vi "Pattern Generator.vi"() -> ()   [LabVIEW 2018]
uses:
  Ctls/Protocol Type.ctl
  Interfaces/File Parser Interface.lvlibp/Interfaces/File Parser Interface/File Parser Interface.lvclass
  Interfaces/Protocol Interface.lvlibp/Interfaces/Protocol Interface/Protocol Interface.lvclass
panel:
  out "error out":errorcluster
  in  "stop":bool
  in  "OK Button":bool
  in  "error in":errorcluster
  in  "PinMap":path
  in  "Frequency(Hz)":dbl=0.1 format="%#_13g"
  in  "Wait between Frames(ms)":dbl=1.0 format="%#_13g"
  in  "NumofCycleRd":u32=1
  in  "Protocol Type":T1
  in  "Config File":path
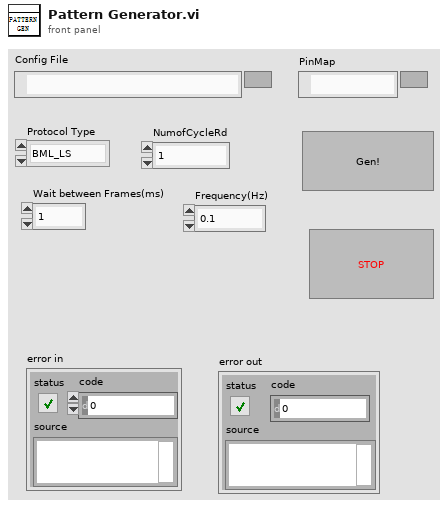
[diagram p1: front panel]
types:
  T1 = typedef "Protocol Type.ctl" = enum16{"BML_LS", "BML_HS", "SPI_3W", "SPI_4W"}
  T2 = cluster{"File Parser Interface.lvclass":refnum<class "File Parser Interface.lvclass">, "Protocol Interface in":refnum<class "Protocol Interface.lvclass">, "Protocol Type":T1, "Config File":path, "Wait between Frames(ms)":dbl, "NumofCycleRd":u32, "PinMap":path, "Frequency(Hz)":dbl}
  T3 = enum16{"init", "wait for input", "Pattern Gen", "error", "end"}
  T4 = typedef "File Parser Interface.lvlibp/Protocol Type.ctl" = enum16{"BML_LS", "BML_HS", "SPI_3W", "SPI_4W"}
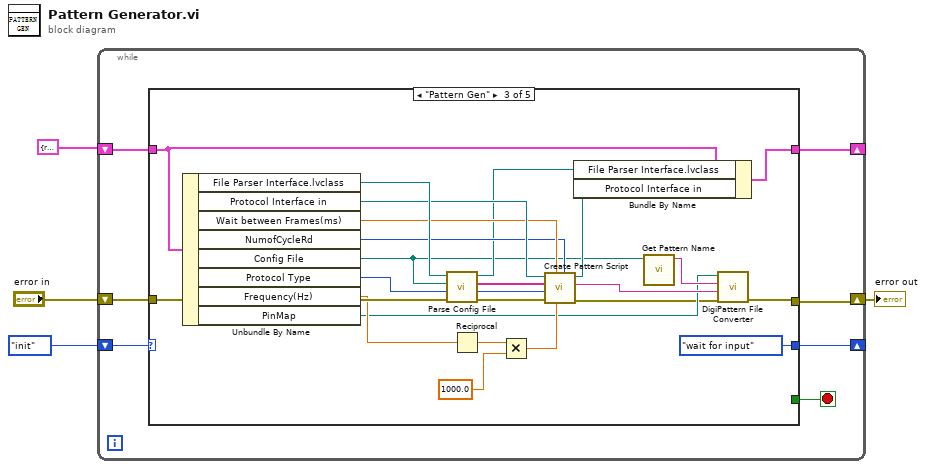
[diagram p0: block diagram]
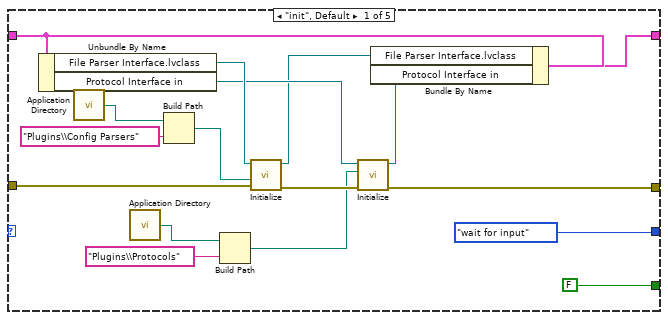
[diagram p2: hidden frame]
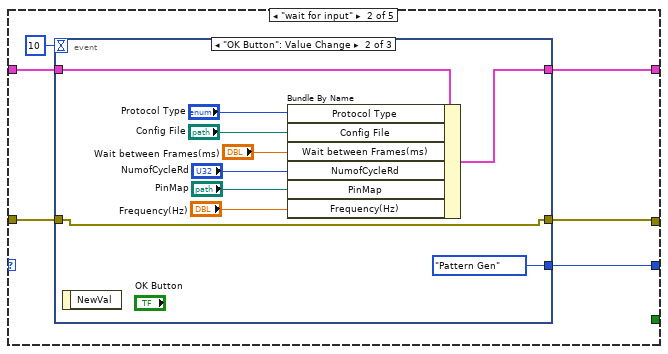
[diagram p3: hidden frame]
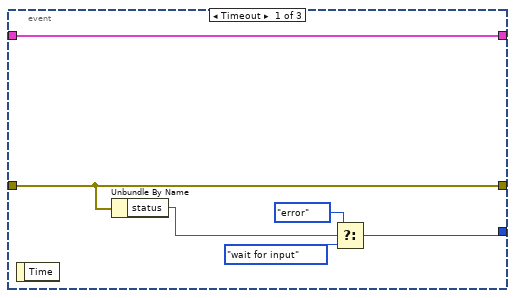
[diagram p4: hidden frame]
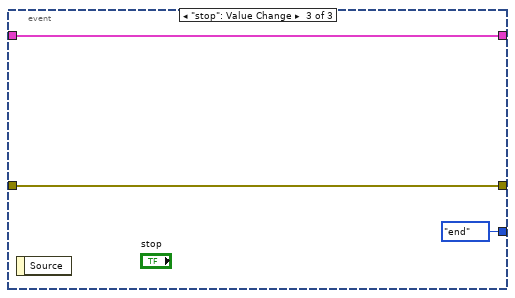
[diagram p5: hidden frame]
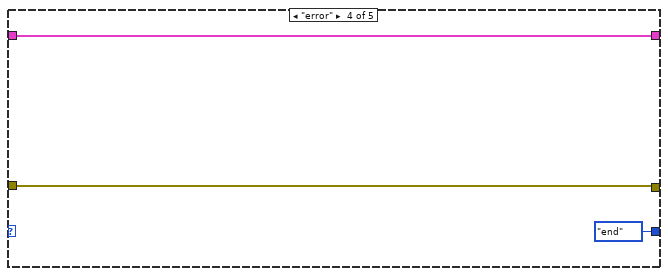
[diagram p6: hidden frame]
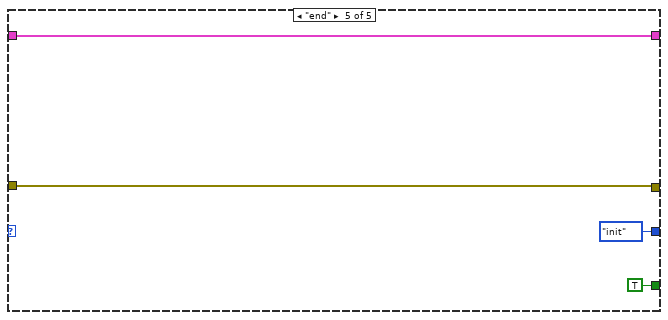
[diagram p7: hidden frame]
diagram:
  n1 = while {
    shift-right: [w10] -> _
    shift-left: T2 {"File Parser Interface.lvclass"=refnum, "Protocol Interface in"=refnum, "Protocol Type"=enum."BML_LS", "Config File"=path "", "Wait between Frames(ms)"=1.0, "NumofCycleRd"=0, "PinMap"=path "", "Frequency(Hz)"=0.0} -> [w11]
    shift-right: [w8] -> w1
    shift-left: "error in" -> [w7]
    shift-right: [w5] -> _
    shift-left: T3."init" -> [w6]
    stop <- w9 stop-if-true
    n2 = case shown="\"Pattern Gen\"" w6 {
      tunnel: w11 -> [w19 w34 w64 w80 w84]
      tunnel: [w16 w33 w61 w80 w84] -> w10
      tunnel: [T3."wait for input" ("f") w29 T3."wait for input" ("f") T3."end" ("f") T3."init" ("f")] -> w5
      tunnel: [FALSE _ _ _ TRUE] -> w9
      tunnel: [w14 w31 w54 w79 w83] -> w8
      tunnel: w7 -> [w13 w32 w77 w79 w83]
      frame "init", Default {
        n3 = Unbundle By Name(w19) -> ("File Parser Interface.lvclass"=w21:refnum<class "File Parser Interface.lvclass">, "Protocol Interface in"=w20:refnum<class "Protocol Interface.lvclass">)
        n4 = call <vilib>:"Application Directory.vi"() -> ("Application Directory"=w27:path)
        n5 = call <vilib>:"Application Directory.vi"() -> ("Application Directory"=w24:path)
        n6 = Build Path(base path=w27, name or relative path="Plugins\\Config Parsers") -> (appended path=w26:path)
        n7 = Build Path(base path=w24, name or relative path="Plugins\\Protocols") -> (appended path=w22:path)
        n8 = call-dynamic "Initialize.vi"("error in (no error)"=w13, "Plugin Folder"=w26, "File Parser Interface in"=w21) -> ("error out"=w25:errorcluster, "File Parser Interface out"=w18:refnum<class "File Parser Interface.lvclass">)  [unwired: 7 in]
        n9 = call "Initialize.vi"("error in (no error)"=w25, "Folder Path"=w22, "Protocol Interface in"=w20) -> ("error out"=w14:errorcluster, "Protocol Interface out"=w17:refnum<class "Protocol Interface.lvclass">)  [unwired: 7 in]
        n10 = Bundle By Name(cluster=w19, "File Parser Interface.lvclass"=w18, "Protocol Interface in"=w17) -> (w16:T2)
      }
      frame "wait for input" {
        n11 = event shown="[1] \"OK Button\": Value Change" {
          selector: _ -> [_ _ _]
          dyn-events: _ -> [_ _ _]
          timeout: 10 -> [_ _ _]
          tunnel: w34 -> [w40 w50 w51]
          tunnel: [w40 w43 w51] -> w33
          tunnel: w32 -> [w39 w42 w53]
          tunnel: [w39 w42 w53] -> w31
          tunnel: [w37 T3."Pattern Gen" T3."end"] -> w29
          event Timeout {
            n12 = event-data() -> ()  [unwired: 1 in, 1 out]
            n13 = Unbundle By Name(w39) -> ("status"=w38:bool)
            n14 = Select(t=T3."error", s=w38, f=T3."wait for input") -> (s? t:f=w37:T3)
          }
          event "OK Button": Value Change {
            n15 = event-data() -> ()  [unwired: 1 in, 1 out]
            n16 = Bundle By Name(cluster=w50, "Protocol Type"="Protocol Type", "Config File"="Config File", "Wait between Frames(ms)"="Wait between Frames(ms)", "NumofCycleRd"="NumofCycleRd", "PinMap"="PinMap", "Frequency(Hz)"="Frequency(Hz)") -> (w43:T2)
          }
          event "stop": Value Change {
            n17 = event-data() -> ()  [unwired: 1 in, 1 out]
          }
        }
      }
      frame "Pattern Gen" {
        n18 = Unbundle By Name(w64) -> ("File Parser Interface.lvclass"=w76:refnum<class "File Parser Interface.lvclass">, "Protocol Interface in"=w74:refnum<class "Protocol Interface.lvclass">, "Wait between Frames(ms)"=w72:dbl, "NumofCycleRd"=w71:u32, "Config File"=w59:path, "Protocol Type"=w69:T1, "Frequency(Hz)"=w68:dbl, "PinMap"=w56:path)
        n19 = call "Parse Config File.vi"("error in (no error)"=w77, "Protocol Type in"=w69, "Config File"=w59, "File Parser Interface in"=w76) -> ("error out"=w75:errorcluster, "Protocol Type out"=w70:T4, "Config Array"=w73:string[], "File Parser Interface out"=w63:refnum<class "File Parser Interface.lvclass">)  [unwired: 4 in]
        n20 = Reciprocal(x=w68) -> (1/x=w67:dbl)
        n21 = Multiply(x=w67, y=1000.0) -> (x*y=w65:dbl)
        n22 = call "Create Pattern Script.vi"("NumofCycleRd"=w71, "Period(ms)"=w65, "Wait(ms)"=w72, "error in (no error)"=w75, "Protocol Type"=w70, "Config Array"=w73, "Protocol Interface in"=w74) -> ("error out"=w55:errorcluster, "Pattern Script out"=w57:string, "Protocol Interface out"=w62:refnum<class "Protocol Interface.lvclass">)  [unwired: 2 in]
        n23 = Bundle By Name(cluster=w64, "File Parser Interface.lvclass"=w63, "Protocol Interface in"=w62) -> (w61:T2)
        n24 = call "Get Pattern Name.vi"("Config file in"=w59) -> ("Pattern Name"=w58:string)  [unwired: 10 in]
        n25 = call "DigiPattern File Converter.vi"("error in (no error)"=w55, "Pattern  Contents"=w57, "Pattern Name"=w58, "PinMap"=w56) -> ("error out"=w54:errorcluster)  [unwired: 7 in]
      }
      frame "error" {
      }
      frame "end" {
      }
    }
  }
  "error out" <- w1
